vi "Init.vi"(5 "Stop User Event in":refnum<user-event>, 7 "Ref FP in":refnum<vi>, 8 "error in (no error)":errorcluster, 9 "Period (ms) in":i64=15, 11 "Keyboard in":refnum<class "Keyboard.lvclass">) -> (0 "error out":errorcluster, 3 "Keyboard out":refnum<class "Keyboard.lvclass">)   [LabVIEW 2024, in "Keyboard.lvclass"]
doc: "MIT Licence\nCopyright (c) 2024 David Grollier"
uses:
  Keyboard.lvclass
  Keyboard.lvclass/Keyboard.ctl
  Input Device.lvclass
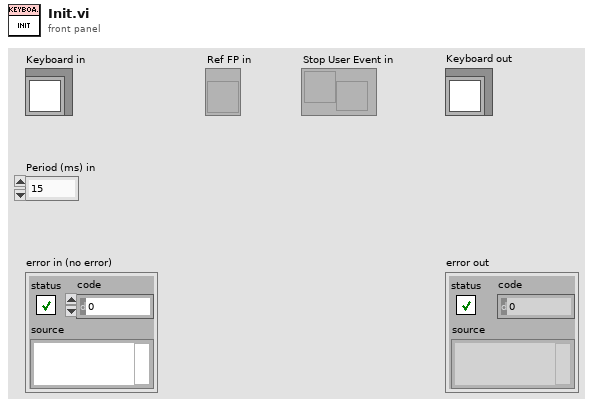
[diagram p1: front panel]
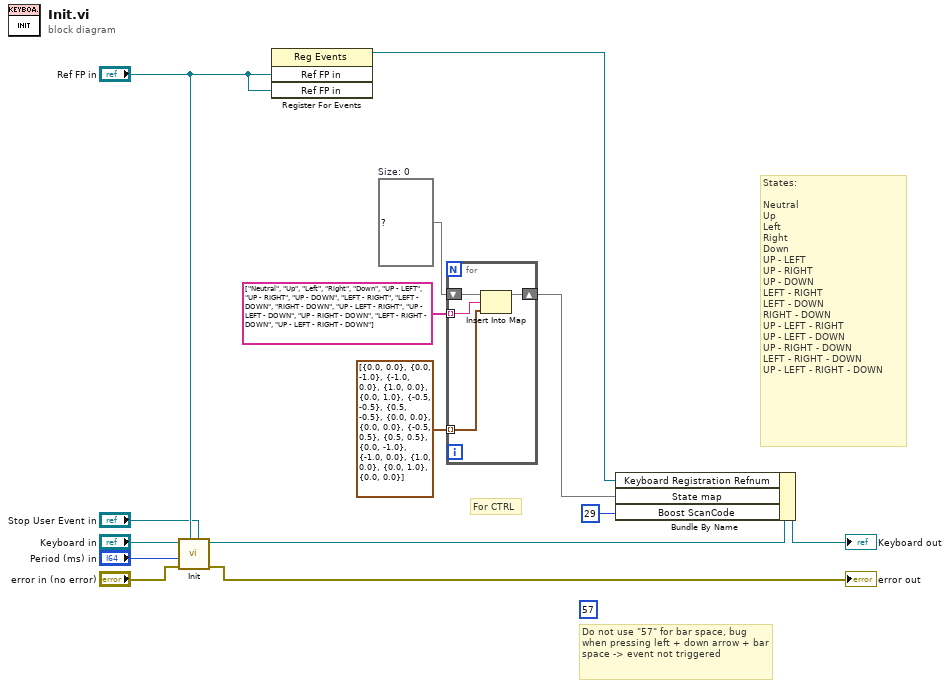
[diagram p0: block diagram]
diagram:
  (unwired) i16 57 ("Boost ScanCode")
  w10 = map{string, cluster{dbl, dbl}} {}  # Size: 0
  # "For CTRL"
  # "Do not use \"57\" for bar space, bug when pressing left + down arrow + bar space -> event not triggered"
  # "States:\n\nNeutral\nUp\nLeft\nRight\nDown\nUP - LEFT\nUP - RIGHT\nUP - DOWN\nLEFT - RIGHT\nLEFT - DOWN\nRIGHT - DOWN\nUP - LEFT - RIGHT\nUP - LEFT - DOWN\nUP - RIGHT - DOWN\nLEFT - RIGHT - DOWN\nUP - LEFT - RIGHT - DOWN"
  n1 = call-parent "Init.vi"("Stop User Event in"="Stop User Event in", "Ref FP in"="Ref FP in", "error in (no error)"="error in (no error)", "Period (ms) in"="Period (ms) in", "Input Device in"="Keyboard in") -> ("error out"=→"error out":errorcluster, "Input Device out"=w14:refnum<class "Keyboard.lvclass">)  [unwired: 5 in]
  n2 = register-events("Ref FP in", "Ref FP in") -> (reference out=w4:refnum<event-registration>)  [unwired: 2 in, 1 out]
  n3 = for {
    shift-right: [w15] -> w7
    shift-left: w10 -> [w18]
    tunnel: string[] ["Neutral", "Up", "Left", "Right", "Down", "UP - LEFT", "UP - RIGHT", "UP - DOWN", "LEFT - RIGHT", "LEFT - DOWN", "RIGHT - DOWN", "UP - LEFT - RIGHT", "UP - LEFT - DOWN", "UP - RIGHT - DOWN", "LEFT - RIGHT - DOWN", "UP - LEFT - RIGHT - DOWN"] -> [w17] mode=indexing
    tunnel: cluster{dbl, dbl}[] [{0.0, 0.0}, {0.0, -1.0}, {-1.0, 0.0}, {1.0, 0.0}, {0.0, 1.0}, {-0.5, -0.5}, {0.5, -0.5}, {0.0, 0.0}, {0.0, 0.0}, {-0.5, 0.5}, {0.5, 0.5}, {0.0, -1.0}, {-1.0, 0.0}, {1.0, 0.0}, {0.0, 1.0}, {0.0, 0.0}] ("Stick out") -> [w16] mode=indexing
    n4 = Insert Into Map(map in=w18, key=w17, value=w16) -> (map out=w15:map{string, cluster{dbl, dbl}})  [unwired: 2 out]
  }
  n5 = Bundle By Name(cluster=w14, "Keyboard Registration Refnum"=w4, "State map"=w7, "Boost ScanCode"=i16 29) -> (→"Keyboard out":refnum<class "Keyboard.lvclass">)
